vi "translateDigitalOutputs.vi"(0 "Controller in":refnum<class "_Controller.lvclass">, 1 "simple_actions":T3, 2 "DO_value (in)":u32, 3 "DO_items (in)":T1[](array[typedef]), 5 "error in (no error)":errorcluster) -> (14 "Controller out":refnum<class "_Controller.lvclass">, 16 "DO_value (out)":u32, 17 "DO_items (out)":T1[](array[typedef]), 19 "error out":errorcluster)   [LabVIEW 2013, in "classes.lvlib" / "_Controller.lvclass"]
uses:
  _Controller.lvclass
  digital_output_item.ctl
  digital_output.ctl
  simple_actions.ctl
  common.lvlib
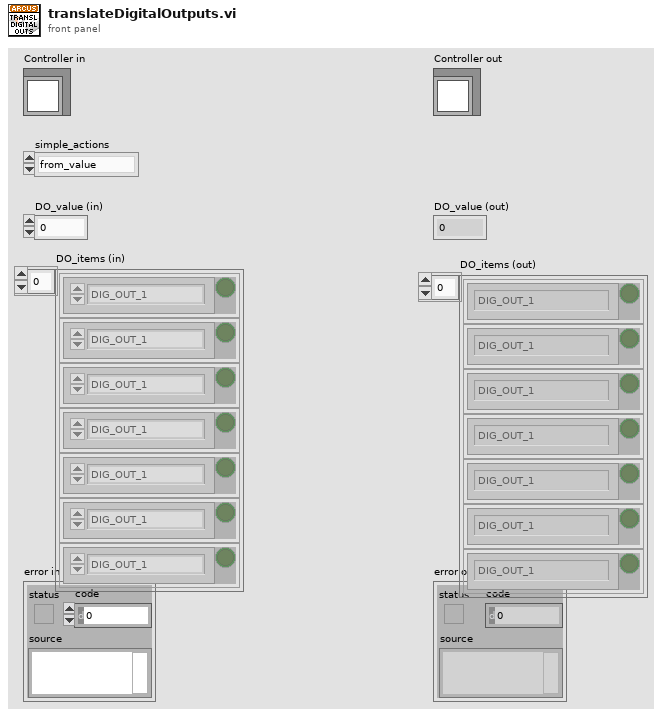
[diagram p1: front panel]
types:
  T1 = typedef "common.lvlib/digital_output_item.ctl" = cluster{"item":T2, "status":bool}
  T2 = typedef "common.lvlib/digital_output.ctl" = enum16{"DIG_OUT_1", "DIG_OUT_2", "DIG_OUT_3", "DIG_OUT_4", "DIG_OUT_5", "DIG_OUT_6", "DIG_OUT_7", "DIG_OUT_8"}
  T3 = typedef "common.lvlib/simple_actions.ctl" = enum16{"from_value", "to_value"}
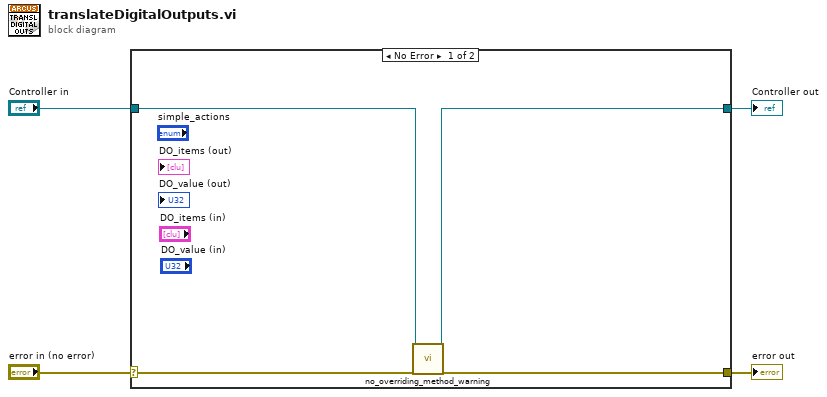
[diagram p0: block diagram]
diagram:
  n1 = case shown="No Error" "error in (no error)" {
    selector: "error in (no error)" -> [w8 w10]
    tunnel: [w7 w10] -> w3
    tunnel: [w5 w9] -> w1
    tunnel: "Controller in" -> [w6 w9]
    frame No Error {
      n2 = call "no_overriding_method_warning.vi"("Controller (in)"=w6, "error in (no error)"=w8) -> ("Controller (out)"=w5:refnum<class "_Controller.lvclass">, "error out"=w7:errorcluster)  [unwired: 15 in, 1 out]
    }
    frame Error {
    }
  }
  "error out" <- w3
  "Controller out" <- w1
